vi "UTL_Load Recipes.vi"(8 "Error in":errorcluster, 9 "Txt Path":path) -> (0 "Error out":errorcluster, 3 "Headers":string[](array[string]), 4 "Sorted 2D table array":string[][](array[string]))   [LabVIEW 2024]
uses:
  <vilib>/Plasmionique/MB Master/MB_Master_Serial/MB_Master_Serial.lvclass
  C:/Program Files (x86)/National Instruments/LabVIEW 2024/vi.lib/Plasmionique/MB Master/MB_Master/MB_Master.lvclass
  Variable global de carga.vi
  <vilib>/Utility/file.llb/Read Delimited Spreadsheet (string).vi
  <vilib>/Plasmionique/MB Master/MB Master.lvlib
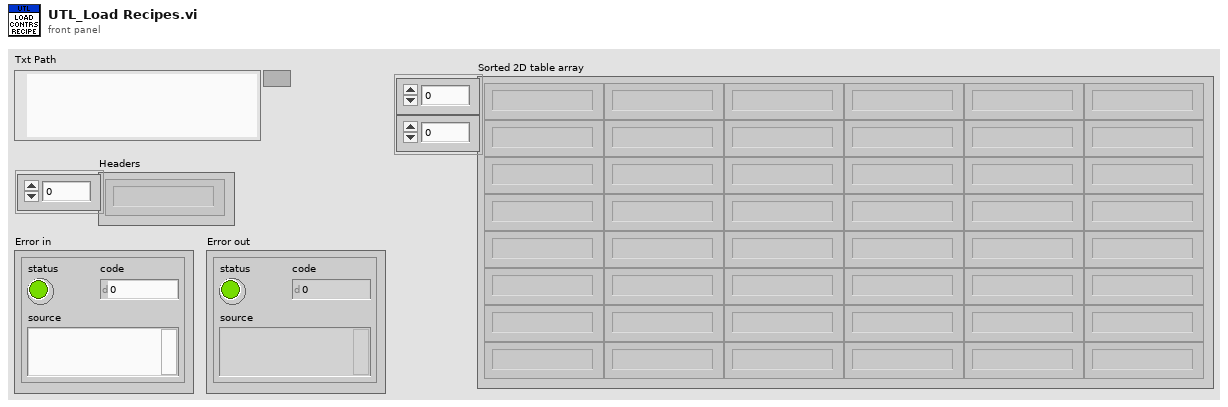
[diagram p1: front panel]
types:
  T1 = typedef "Control 2.ctl" = refnum<class "MB_Master_Serial.lvclass">[]
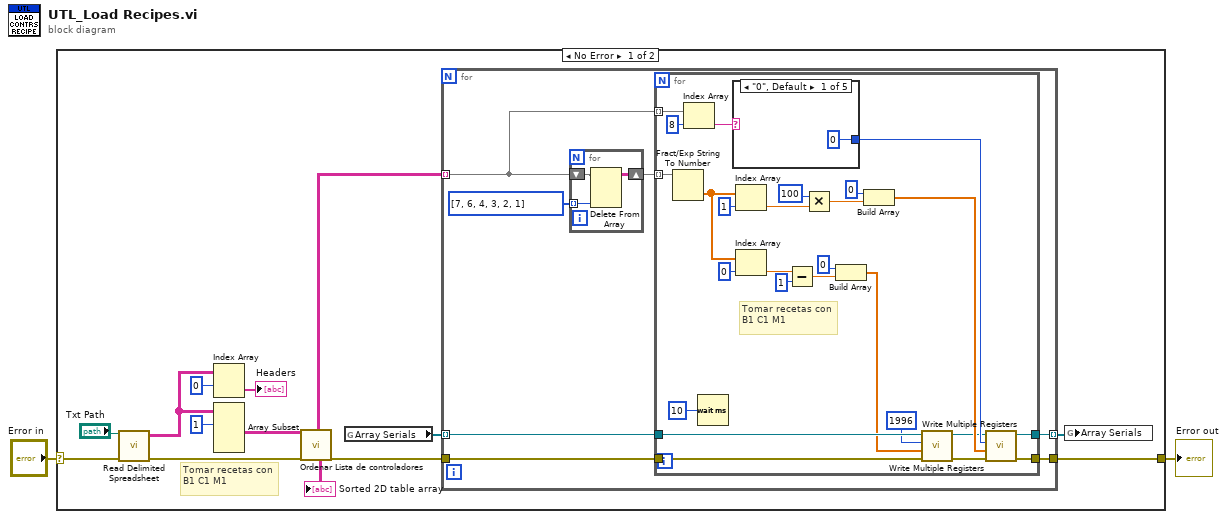
[diagram p0: block diagram]
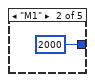
[diagram p2: hidden frame]
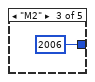
[diagram p3: hidden frame]
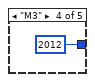
[diagram p4: hidden frame]
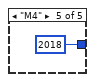
[diagram p5: hidden frame]
diagram:
  n1 = case shown="No Error" "Error in" {
    selector: "Error in" -> [w6 w58]
    tunnel: [w4 w58] -> w1
    frame No Error {
      # "Tomar recetas con B1 C1 M1"
      n2 = call-poly <vilib>:"Read Delimited Spreadsheet.vi"("file path (dialog if empty)"="Txt Path", "error in (no error)"=w6) -> ("all rows"=w9:string[][], "error out"=w10:errorcluster)  [unwired: 8 in, 4 out]
      n3 = Index Array(array=w9, index (row)=0) -> (element=→"Headers":string[])  [unwired: 1 in]
      n4 = Array Subset(array=w9, index (row)=1 ("index")) -> (w12:string[][])  [unwired: 3 in]
      n5 = call "Ordenar Lista de controladores.vi"("subarray"=w12, "error in (no error)"=w10) -> ("3D Ordered array"=w5:string[][][], "Sorted 2D table array"=→"Sorted 2D table array":string[][], "error out"=w11:errorcluster)  [unwired: 15 in]
      n6 = global read "Variable global de carga.vi" "Array Serials"() -> (w8:T1)
      n7 = for {
        tunnel: w5 -> [w21] mode=indexing
        tunnel: w11 -> [w19]
        tunnel: [w17] -> w4
        tunnel: w8 -> [w20] mode=indexing
        tunnel: [w18] -> w7 mode=indexing
        n8 = for {
          tunnel: i32[] [7, 6, 4, 3, 2, 1] ("y") -> [w24] mode=indexing
          shift-right: [w25] -> w22
          shift-left: w21 -> [w26]
          n9 = Delete From Array(array=w26, index (col)=w24) -> (array with subset deleted=w25:string[][])  [unwired: 2 in, 1 out]
        }
        n10 = for {
          tunnel: w19 -> [w51]
          tunnel: [w52] -> w17
          tunnel: w20 -> [w50]
          tunnel: [w49] -> w18
          tunnel: w22 -> [w29] mode=indexing
          tunnel: w21 -> [w28] mode=indexing
          # "Tomar recetas con B1 C1 M1"
          n11 = Fract/Exp String To Number(string=w29) -> (number=w30:dbl[])  [unwired: 3 in, 1 out]
          n12 = Index Array(array=w28, index=8) -> (element=w48:string)
          n13 = Wait (ms)(milliseconds to wait=u32 10) -> ()  [unwired: 1 out]
          n14 = case shown="\"0\", Default" w48 {
            tunnel: [0 u16 2000 2006 2012 2018] -> w37
            frame "0", Default {
            }
            frame "M1" {
            }
            frame "M2" {
            }
            frame "M3" {
            }
            frame "M4" {
            }
          }
          n15 = Index Array(array=w30, index=1) -> (element=w42:dbl)
          n16 = Index Array(array=w30, index=0) -> (element=w31:dbl)
          n17 = Subtract(x=w31, y=1) -> (x-y=w44:dbl)
          n18 = Multiply(x=100, y=w42) -> (x*y=w40:dbl)
          n19 = Build Array(0, w44) -> (w32:dbl[])
          n20 = Build Array(0, w40) -> (w38:dbl[])
          n21 = call <vilib>:"Write Multiple Registers.vi"("error in (no error)"=w51, "values"=w32, "starting address"=u16 1996, "MB session in"=w50) -> ("error out"=w36:errorcluster, "MB session out"=w35:refnum<class "MB_Master_Serial.lvclass">)  [unwired: 6 in]
          n22 = call <vilib>:"Write Multiple Registers.vi"("error in (no error)"=w36, "values"=w38, "starting address"=w37, "MB session in"=w35) -> ("error out"=w52:errorcluster, "MB session out"=w49:refnum<class "MB_Master_Serial.lvclass">)  [unwired: 6 in]
        }
      }
      n23 = global write "Variable global de carga.vi" "Array Serials"(w7) -> ()
    }
    frame Error {
    }
  }
  "Error out" <- w1
